vi "Parse Time.vi"(11 "parse time":string) -> (3 "time (HH:MM:SS)":dbl format="%<%H:%M:%S>t")   [LabVIEW 2019, in "Pet Feeder.lvlib"]
uses:
  Pet Feeder.lvlib
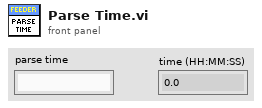
[diagram p1: front panel]
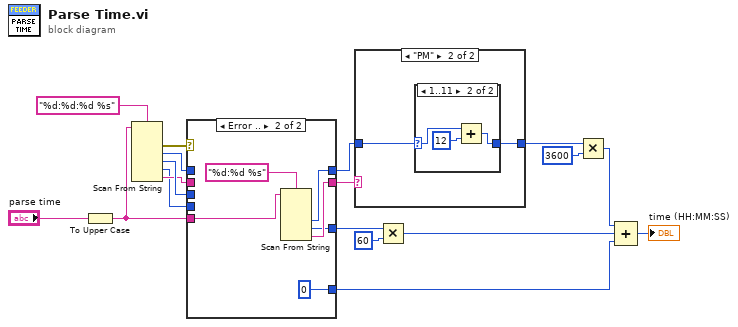
[diagram p0: block diagram]
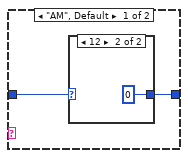
[diagram p3: hidden frame]
diagram:
  n1 = To Upper Case(1:"parse time") -> (0:w1:string)
  n2 = Scan From String(format string="%d:%d:%d %s", input string=w1) -> (error out=w7:errorcluster, output 1=w6:i32, output 2=w5:i32, output 3=w2:i32, output 4=w4:string)  [unwired: 6 in, 2 out]
  n3 = case shown="Error .." w7 {
    tunnel: [w22 w27] -> w17
    tunnel: [w20 w26] -> w16
    tunnel: [w21 w25] -> w13
    tunnel: w6 -> [w22 _]
    tunnel: w5 -> [w21 _]
    tunnel: w4 -> [w20 _]
    tunnel: [w19 0 ("y")] -> w3
    tunnel: w2 -> [w19 _]
    tunnel: w1 -> [_ w23]
    frame No Error {
    }
    frame Error {
      n4 = Scan From String(format string="%d:%d %s", input string=w23) -> (output 1=w27:i32, output 2=w25:i32, output 3=w26:string)  [unwired: 5 in, 3 out]
    }
  }
  n5 = case shown="\"PM\"" w16 {
    tunnel: w17 -> [w30 w34]
    tunnel: [w29 w33] -> w15
    frame "AM", Default {
      n6 = case shown="12" w30 {
        selector: w30 -> [w31 _]
        tunnel: [w31 0] -> w29
        frame Default {
        }
        frame 12 {
        }
      }
    }
    frame "PM" {
      n7 = case shown="1..11" w34 {
        selector: w34 -> [w35 w38]
        tunnel: [w35 w36] -> w33
        frame Default {
        }
        frame 1..11 {
          n8 = Add(x=w38, y=12) -> (x+y=w36:i32)
        }
      }
    }
  }
  n9 = Multiply(x=w13, y=60) -> (x*y=w10:i32)
  n10 = Multiply(x=w15, y=3600) -> (x*y=w11:i32)
  n11 = Compound Arithmetic op=ADD(w11, w10, w3) -> (→"time (HH:MM:SS)":i32)
